vi "ForwardsPickup.vi"   [LabVIEW 2014]
types:
  T1 = cluster{"Rate":dbl, "Direction":bool, "Stopped":bool}[]
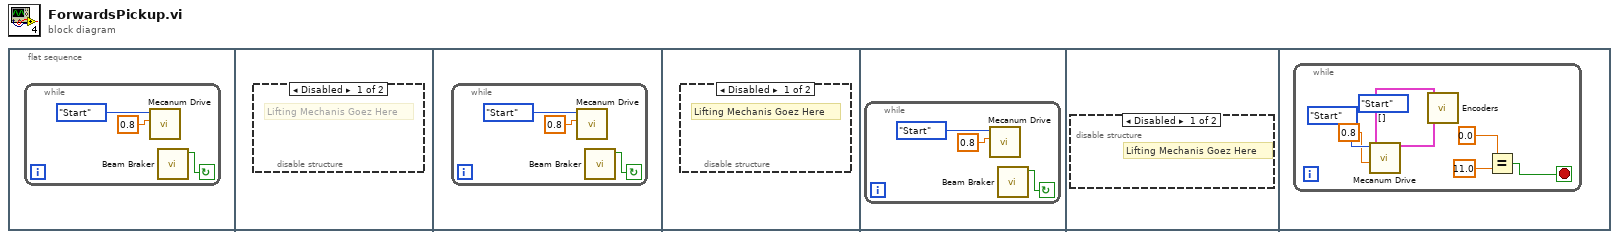
[diagram p0: block diagram]
diagram:
  n1 = flat-sequence {
    frame #0 {
      n2 = while {
        stop <- w1 continue-if-true
        n3 = call "Mecanum Drive.vi"("Forward/Backward"=0.8, "Mode"=enum8{"Start", "Run", "Finish"}."Start") -> ()  [unwired: 10 in]
        n4 = call "Beam Braker.vi"() -> ("Boolean"=w1:bool)  [unwired: 11 in]
      }
    }
    frame #1 {
      n5 = disable-structure shown="Disabled" {
        frame Disabled {
          # "Lifting Mechanis Goez Here"
        }
        frame Enabled {
        }
      }
    }
    frame #2 {
      n6 = while {
        stop <- w4 continue-if-true
        n7 = call "Mecanum Drive.vi"("Forward/Backward"=0.8, "Mode"=enum8{"Start", "Run", "Finish"}."Start") -> ()  [unwired: 10 in]
        n8 = call "Beam Braker.vi"() -> ("Boolean"=w4:bool)  [unwired: 11 in]
      }
    }
    frame #3 {
      n9 = disable-structure shown="Disabled" {
        frame Disabled {
          # "Lifting Mechanis Goez Here"
        }
        frame Enabled {
        }
      }
    }
    frame #4 {
      n10 = while {
        stop <- w7 continue-if-true
        n11 = call "Mecanum Drive.vi"("Forward/Backward"=0.8, "Mode"=enum8{"Start", "Run", "Finish"}."Start") -> ()  [unwired: 10 in]
        n12 = call "Beam Braker.vi"() -> ("Boolean"=w7:bool)  [unwired: 11 in]
      }
    }
    frame #5 {
      n13 = disable-structure shown="Disabled" {
        frame Disabled {
          # "Lifting Mechanis Goez Here"
        }
        frame Enabled {
        }
      }
    }
    frame #6 {
      n14 = while {
        stop <- w10 stop-if-true
        (unwired) T1 [] ("Encoder")
        n15 = call "Mecanum Drive.vi"("Strafe"=0.8, "Mode"=enum8{"Start", "Run", "Finish"}."Start") -> ()  [unwired: 10 in]
        n16 = call "Encoders.vi"("Mode"=enum8{"Start", "Run", "Finish"}."Start") -> ()  [unwired: 3 in, 1 out]
        n17 = Equal?(x=0.0 ("Distance"), y=11.0) -> (x = y?=w10:bool)
      }
    }
  }
